vi "Crossover v1.vi"(10 "Path In 2":T1={"Distance"=0.0, "Tour"=[1, 14, 13, 12, 7, 6, 15, 5, 11, 9, 10, 16, 3, 2, 4, 8, 1]}, 11 "Path In 1":T1={"Distance"=0.0, "Tour"=[1, 14, 13, 12, 7, 6, 15, 5, 11, 9, 10, 16, 3, 2, 4, 8, 1]}) -> (2 "Path Out 2":T1={"Distance"=0.0, "Tour"=[68, 82, 14, 66, 38, 76, 91, 89, 87, 84, 25, 25, 88]}, 3 "Path Out 1":T1={"Distance"=0.0, "Tour"=[68, 82, 14, 66, 38, 76, 91, 89, 87, 84, 25, 25, 88]})   [LabVIEW 2015, in "TSP Library.lvlib"]
uses:
  TSP Library.lvlib
  TypeDef/Path.ctl
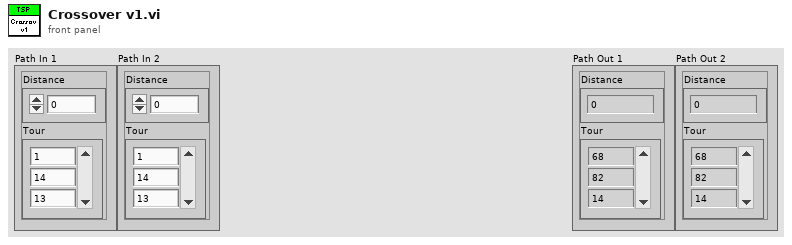
[diagram p1: front panel]
types:
  T1 = typedef "TSP Library.lvlib/Path.ctl" = cluster{"Distance":dbl, "Tour":u16[]}
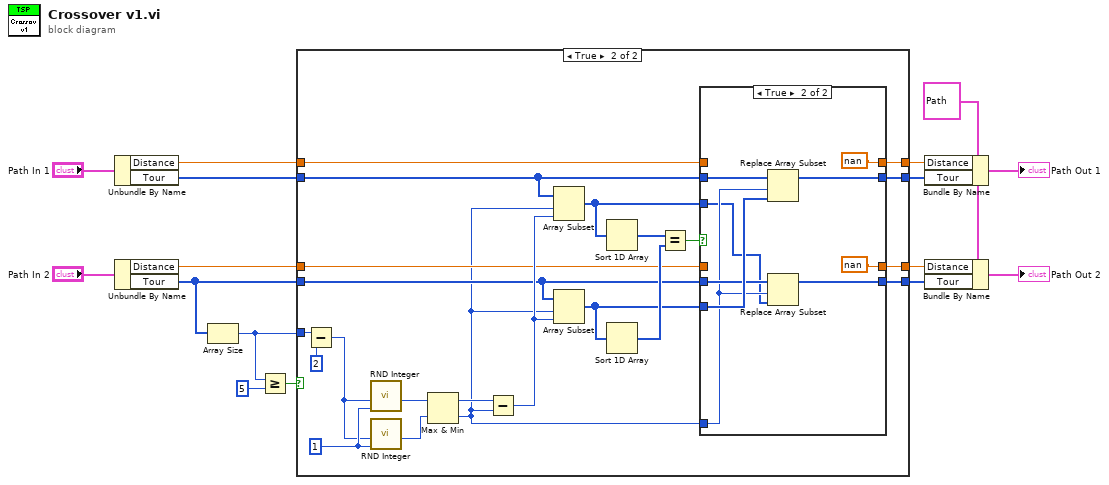
[diagram p0: block diagram]
diagram:
  w9 = T1 {"Distance"=0.0, "Tour"=[68, 82, 14, 66, 38, 76, 91, 89, 87, 84, 25, 25, 88]} ("Path In 1")
  n1 = Unbundle By Name("Path In 1") -> ("Distance"=w11:dbl, "Tour"=w12:u16[])
  n2 = Unbundle By Name("Path In 2") -> ("Distance"=w13:dbl, "Tour"=w14:u16[])
  n3 = Array Size(array=w14) -> (size(s)=w2:i32)
  n4 = Greater Or Equal?(x=w2, y=5) -> (x >= y?=w3:bool)
  n5 = case shown="True" w3 {
    tunnel: w2 -> [_ w42]
    tunnel: w14 -> [w17 w34]
    tunnel: w13 -> [w18 w33]
    tunnel: w12 -> [w19 w32]
    tunnel: w11 -> [w20 w31]
    tunnel: [w19 w30] -> w7
    tunnel: [w17 w29] -> w6
    tunnel: [w18 w28] -> w5
    tunnel: [w20 w27] -> w4
    frame False {
    }
    frame True {
      w22 = 1 ("Min")
      n6 = Subtract(x=w42, y=2) -> (x-y=w21:i32)
      n7 = call "RND Integer.vi"("Min"=w22, "Max"=w21) -> ("RND Integer"=w24:i32)  [unwired: 9 in]
      n8 = call "RND Integer.vi"("Min"=w22, "Max"=w21) -> ("RND Integer"=w23:i32)  [unwired: 9 in]
      n9 = Max & Min(x=w24, y=w23) -> (max(x,y)=w41:i32, min(x,y)=w26:i32)
      n10 = Subtract(x=w41, y=w26) -> (x-y=w40:i32)
      n11 = Array Subset(array=w32, index=w26, length=w40) -> (w36:u16[])
      n12 = Array Subset(array=w34, index=w26, length=w40) -> (w35:u16[])
      n13 = Sort 1D Array(array=w36) -> (sorted array=w39:u16[])
      n14 = Sort 1D Array(array=w35) -> (sorted array=w38:u16[])
      n15 = Equal?(x=w39, y=w38) -> (x = y?=w37:bool)
      n16 = case shown="True" w37 {
        tunnel: w36 -> [_ w49]
        tunnel: w35 -> [_ w54]
        tunnel: w34 -> [w45 w51]
        tunnel: w33 -> [w44 _]
        tunnel: w32 -> [w46 w55]
        tunnel: w31 -> [w43 _]
        tunnel: [w46 w53] -> w30
        tunnel: [w45 w52] -> w29
        tunnel: [w44 nan ("Distance")] -> w28
        tunnel: [w43 nan ("Distance")] -> w27
        tunnel: w26 -> [_ w50]
        frame False {
        }
        frame True {
          n17 = Replace Array Subset(array=w55, new element=w54, index=w50) -> (w53:u16[])
          n18 = Replace Array Subset(array=w51, new element=w49, index=w50) -> (w52:u16[])
        }
      }
    }
  }
  n19 = Bundle By Name(cluster=w9, "Distance"=w4, "Tour"=w7) -> (→"Path Out 1":T1)
  n20 = Bundle By Name(cluster=w9, "Distance"=w5, "Tour"=w6) -> (→"Path Out 2":T1)
